vi "WPI_ADI_IMU_Open.vi"(8 "error in":errorcluster, 9 "AHRS Algorithm":enum16{"Complementary", "Madgwick"}(ring), 10 "Yaw Axis":enum16{"X", "Y", "Z"}(ring)=enum."Z", 11 "SPI Chip Select":T3=enum."SPI MXP") -> (0 "error out":errorcluster, 3 "ADI IMU Interrupt DevRef":T1={"SimpleGyroDevRef"={"DevStatus"={"status"=FALSE, "code"=0, "source"=""}, "Handle"=0, "SPI Bus"=enum."SPI On-Board, CS0", "Device Found"=FALSE, "Sample Rate"=0.0, "Device Ready"=FALSE, "Yaw Axis"=enum."Z", "AHRS Algorithm"=enum."Complementary"}, "InterruptRef"={"DevStatus"={"status"=FALSE, "code"=0, "source"=""}, "InterruptIndex"=enum."0"}} {"SimpleGyroDevRef"."Sample Rate" min=0.25 max=100.0 step=0.25})   [LabVIEW 2015, in "FRC ADI MXP IMU.lvlib"]
doc: "Initiates communication between an Analog Devices MXP IMU and the RoboRIO."
uses:
  FRC ADI MXP IMU.lvlib
  <vilib>/Rock Robotics/SystemInterfaces/spilib/spi_bus.ctl
  WPI_AnalogDevicesIMUInterruptDevRef.ctl
  WPI_AnalogDevicesIMUDevRef.ctl
  <vilib>/Rock Robotics/WPI/Interrupt/WPI_InterruptRef.ctl
  <vilib>/Rock Robotics/SystemInterfaces/Interrupt/FPGA_InterruptIndex.ctl
  <vilib>/Rock Robotics/WPI/SPI/WPI_SPIMode.ctl
  <vilib>/Rock Robotics/SystemInterfaces/DIO/FPGA_DIOChannel.ctl
  WPI_IMU_ADIS16448_Registers.ctl
  <vilib>/Rock Robotics/WPI/Counter/WPI_CounterDigitalInputToDigitalSource.vi
  <vilib>/Rock Robotics/SystemInterfaces/CounterEncoderSourceConvertion/FPGA_CounterEncoderSourceConvertionLVSourceTypeToFPGAType.vi
  <vilib>/Rock Robotics/WPI/Interrupt/WPI_InterruptCache.vi
  <vilib>/Rock Robotics/SystemInterfaces/Interrupt/FPGA_InterruptWriteConfiguration.vi
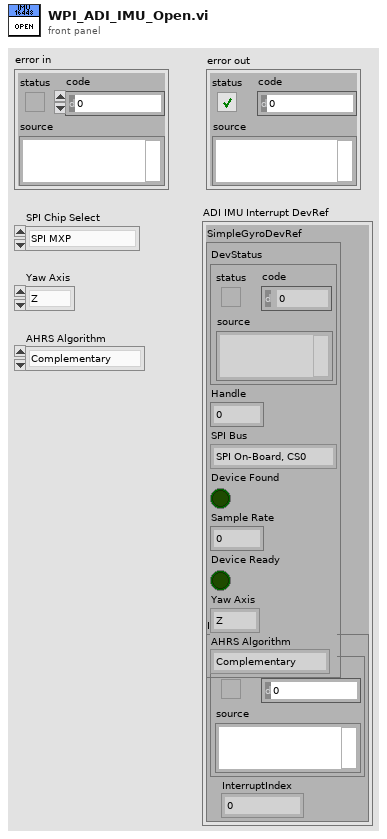
[diagram p1: front panel]
types:
  T1 = typedef "FRC ADI MXP IMU.lvlib/WPI_AnalogDevicesIMUInterruptDevRef.ctl" = cluster{"SimpleGyroDevRef":T2, "InterruptRef":T4}
  T2 = typedef "FRC ADI MXP IMU.lvlib/WPI_AnalogDevicesIMUDevRef.ctl" = cluster{"DevStatus":errorcluster, "Handle":i32, "SPI Bus":T3, "Device Found":bool, "Sample Rate":dbl, "Device Ready":bool, "Yaw Axis":enum16{"X", "Y", "Z"}, "AHRS Algorithm":enum16{"Complementary", "Madgwick"}}
  T3 = typedef "spi_bus.ctl" = enum16{"SPI On-Board, CS0", "SPI On-Board, CS1", "SPI On-Board, CS2", "SPI On-Board, CS3", "SPI MXP", "Invalid"}
  T4 = typedef "WPI_InterruptRef.ctl" = cluster{"DevStatus":errorcluster, "InterruptIndex":T5}
  T5 = typedef "FPGA_InterruptIndex.ctl" = enum8{"0", "1", "2", "3", "4", "5", "6", "7", "Invalid"}
  T6 = typedef "FPGA_DIOChannel.ctl" = enum8{"DIO 0", "DIO 1", "DIO 2", "DIO 3", "DIO 4", "DIO 5", "DIO 6", "DIO 7", "DIO 8", "DIO 9", "DIO MXP 0", "DIO MXP 1", "DIO MXP 2", "DIO MXP 3", "DIO MXP 4", "DIO MXP 5", "DIO MXP 6", "DIO MXP 7", "DIO MXP 8", "DIO MXP 9", "DIO MXP 10", "DIO MXP 11", "DIO MXP 12", "DIO MXP 13", "DIO MXP 14", "DIO MXP 15", "Invalid"}
  T7 = typedef "WPI_SPIMode.ctl" = enum16{"Mode 0 (Clk Idle Low,Sample on Leading)", "Mode 1 (Clk Idle Low,Sample on Trailing)", "Mode 2 (Clk Idle High,Sample on Leading)", "Mode 3 (Clk Idle High,Sample on Trailing)"}
  T8 = typedef "FRC ADI MXP IMU.lvlib/WPI_IMU_ADIS16448_Registers.ctl" = u8
  T9 = typedef "WPI_SPIDevRef.ctl" = cluster{"DevStatus":errorcluster, "Handle":i32, "SPI Bus":T3}
  T10 = typedef "WPI_DigitalInputDevRef.ctl" = cluster{"DevStatus":errorcluster, "DIO Channel":T6}
  T11 = typedef "FPGA_CounterEncoderSourceConvertionLVSourceType.ctl" = cluster{"DevStatus":errorcluster, "AnalogTriggerMode?":bool, "DigitalMode":cluster{"DIO Channel":T12}, "AnalogTriggerMode":cluster{"AnalogTriggerIndex":T13, "OutputType":T14}}
  T12 = typedef "FPGA_DIODigitalSourceChannel.ctl" = enum8{"DIO 0", "DIO 1", "DIO 2", "DIO 3", "DIO 4", "DIO 5", "DIO 6", "DIO 7", "DIO 8", "DIO 9", "DIO MXP 0", "DIO MXP 1", "DIO MXP 2", "DIO MXP 3", "DIO MXP 4", "DIO MXP 5", "DIO MXP 6", "DIO MXP 7", "DIO MXP 8", "DIO MXP 9", "DIO MXP 10", "DIO MXP 11", "DIO MXP 12", "DIO MXP 13", "DIO MXP 14", "DIO MXP 15", "Disabled"}
  T13 = typedef "FPGA_AnalogTriggerIndex.ctl" = enum8{"Trig 0", "Trig 1", "Trig 2", "Trig 3", "Trig 4", "Trig 5", "Trig 6", "Trig 7", "Invalid"}
  T14 = typedef "FPGA_AnalogTriggerOutType.ctl" = enum16{"InWindow", "TriggerState", "Rising", "Falling"}
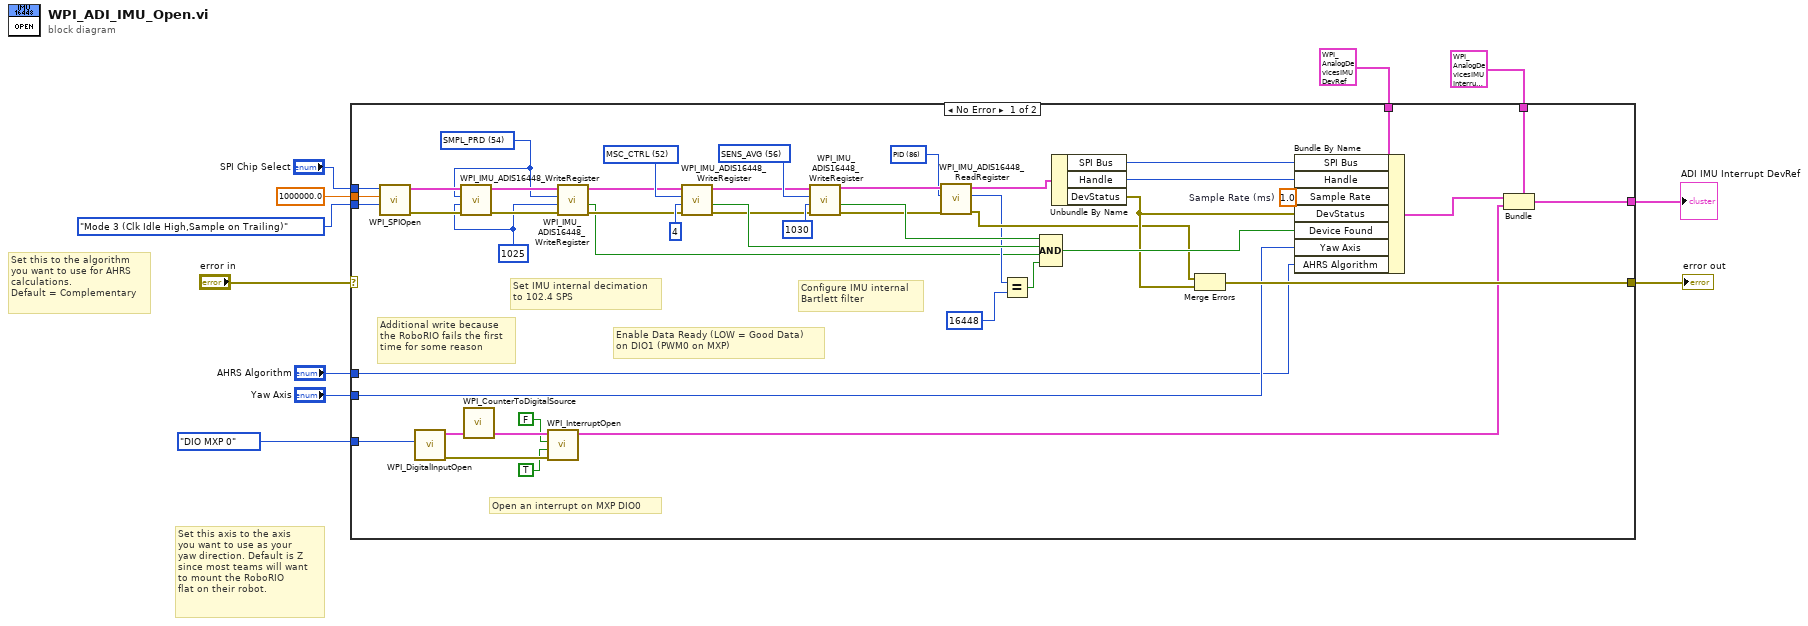
[diagram p0: block diagram]
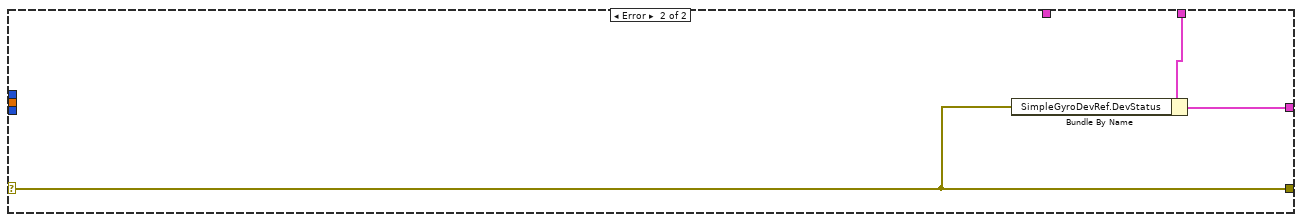
[diagram p2: hidden frame]
diagram:
  # "Set this to the algorithm\nyou want to use for AHRS\ncalculations. \nDefault = Complementary"
  # "Set this axis to the axis\nyou want to use as your\nyaw direction. Default is Z\nsince most teams will want \nto mount the RoboRIO\nflat on their robot."
  n1 = case shown="No Error" "error in" {
    selector: "error in" -> [_ w60]
    tunnel: "SPI Chip Select" -> [w58 _]
    tunnel: 1000000.0 ("Clock Rate (Hz)") -> [w57 _]
    tunnel: WPI_SPIMode."Mode 3 (Clk Idle High,Sample on Trailing)" ("Mode (3)") -> [w56 _]
    tunnel: [w46 w60] -> w7
    tunnel: T2 {"DevStatus"={"status"=FALSE, "code"=0, "source"=""}, "Handle"=0, "SPI Bus"=enum."SPI On-Board, CS0", "Device Found"=FALSE, "Sample Rate"=0.0, "Device Ready"=FALSE, "Yaw Axis"=enum."Z", "AHRS Algorithm"=enum."Complementary"} ("SimpleGyroDevRef 2") -> [w55 _]
    tunnel: [w33 w59] -> w3
    tunnel: T1 {"SimpleGyroDevRef"={"DevStatus"={"status"=FALSE, "code"=0, "source"=""}, "Handle"=0, "SPI Bus"=enum."SPI On-Board, CS0", "Device Found"=FALSE, "Sample Rate"=0.0, "Device Ready"=FALSE, "Yaw Axis"=enum."Z", "AHRS Algorithm"=enum."Complementary"}, "InterruptRef"={"DevStatus"={"status"=FALSE, "code"=0, "source"=""}, "InterruptIndex"=enum."0"}} ("output cluster") -> [w32 w61]
    tunnel: FPGA_DIOChannel."DIO MXP 0" ("DIO Channel") -> [w31 _]
    tunnel: "Yaw Axis" -> [w13 _]
    tunnel: "AHRS Algorithm" -> [w12 _]
    frame No Error {
      w27 = T8 86 items=["SMPL_PRD"=54, "SENS_AVG"=56, "MSC_CTRL"=52, "ERROR_FLAGS"=60, "TEMP"=44, "BARO"=40, "Z_MAG"=36, "Y_MAG"=32, "X_MAG"=28, "Z_ACCEL"=24, "Y_ACCEL"=20, "X_ACCEL"=16, "Z_GYRO"=12, "Y_GYRO"=8, "X_GYRO"=4, "PID"=86] ("ADIS16448 Register")
      w52 = 1.0  # Sample Rate (ms)
      w45 = T8 56 items=["SMPL_PRD"=54, "SENS_AVG"=56, "MSC_CTRL"=52, "ERROR_FLAGS"=60, "TEMP"=44, "BARO"=40, "Z_MAG"=36, "Y_MAG"=32, "X_MAG"=28, "Z_ACCEL"=24, "Y_ACCEL"=20, "X_ACCEL"=16, "Z_GYRO"=12, "Y_GYRO"=8, "X_GYRO"=4, "PID"=86] ("ADIS16448 Register")
      w51 = T8 52 items=["SMPL_PRD"=54, "SENS_AVG"=56, "MSC_CTRL"=52, "ERROR_FLAGS"=60, "TEMP"=44, "BARO"=40, "Z_MAG"=36, "Y_MAG"=32, "X_MAG"=28, "Z_ACCEL"=24, "Y_ACCEL"=20, "X_ACCEL"=16, "Z_GYRO"=12, "Y_GYRO"=8, "X_GYRO"=4, "PID"=86] ("ADIS16448 Register")
      w17 = u16 1025 ("Data")
      w16 = T8 54 items=["SMPL_PRD"=54, "SENS_AVG"=56, "MSC_CTRL"=52, "ERROR_FLAGS"=60, "TEMP"=44, "BARO"=40, "Z_MAG"=36, "Y_MAG"=32, "X_MAG"=28, "Z_ACCEL"=24, "Y_ACCEL"=20, "X_ACCEL"=16, "Z_GYRO"=12, "Y_GYRO"=8, "X_GYRO"=4, "PID"=86] ("ADIS16448 Register")
      # "Open an interrupt on MXP DIO0"
      # "Additional write because\nthe RoboRIO fails the first\ntime for some reason"
      # "Configure IMU internal\nBartlett filter"
      # "Enable Data Ready (LOW = Good Data) \non DIO1 (PWM0 on MXP)"
      # "Set IMU internal decimation\nto 102.4 SPS"
      n2 = call <vilib>:"WPI_SPIOpen.vi"("Mode (3)"=w56, "Clock Rate (Hz)"=w57, "SPI Bus"=w58) -> ("error out"=w18:errorcluster, "SPIDevRef"=w21:T9)  [unwired: 7 in]
      n3 = call <vilib>:"WPI_DigitalInputOpen.vi"("DIO Channel"=w31) -> ("error out"=w38:errorcluster, "DigitalInputDevRef"=w40:T10)  [unwired: 9 in]
      n4 = call "WPI_IMU_ADIS16448_WriteRegister.vi"("error in (no error)"=w18, "Data"=w17, "ADIS16448 Register"=w16, "SPIDevRef in"=w21) -> ("error out"=w19:errorcluster, "SPIDevRef out"=w20:T9)  [unwired: 4 in, 2 out]
      n5 = call-poly <vilib>:"WPI_CounterToDigitalSource.vi"("DigitalInputDevRef"=w40) -> ("Digital Source"=w39:T11)  [unwired: 6 in]
      n6 = call <vilib>:"WPI_InterruptOpen.vi"("error in (no error)"=w38, "Falling Edge"=TRUE, "Rising Edge"=FALSE, "Source"=w39) -> ("InterruptRef"=w35:T4)  [unwired: 6 in, 1 out]
      n7 = call "WPI_IMU_ADIS16448_WriteRegister.vi"("error in (no error)"=w19, "Data"=w17, "ADIS16448 Register"=w16, "SPIDevRef in"=w20) -> ("error out"=w24:errorcluster, "Write OK?"=w14:bool, "SPIDevRef out"=w25:T9)  [unwired: 4 in, 1 out]
      n8 = call "WPI_IMU_ADIS16448_WriteRegister.vi"("error in (no error)"=w24, "Data"=u16 4, "ADIS16448 Register"=w51, "SPIDevRef in"=w25) -> ("error out"=w42:errorcluster, "Write OK?"=w48:bool, "SPIDevRef out"=w43:T9)  [unwired: 4 in, 1 out]
      n9 = call "WPI_IMU_ADIS16448_WriteRegister.vi"("error in (no error)"=w42, "Data"=u16 1030, "ADIS16448 Register"=w45, "SPIDevRef in"=w43) -> ("error out"=w28:errorcluster, "Write OK?"=w41:bool, "SPIDevRef out"=w29:T9)  [unwired: 4 in, 1 out]
      n10 = call "WPI_IMU_ADIS16448_ReadRegister.vi"("error in (no error)"=w28, "Register"=w27, "SPIDevRef in"=w29) -> ("error out"=w26:errorcluster, "Register Value"=w23:u16, "SPIDevRef out"=w30:T9)  [unwired: 6 in]
      n11 = Equal?(x=w23, y=u16 16448) -> (x = y?=w15:bool)
      n12 = Compound Arithmetic op=AND(w41, w48, w14, w15) -> (w49:bool)
      n13 = Unbundle By Name(w30) -> ("SPI Bus"=w54:T3, "Handle"=w53:i32, "DevStatus"=w47:errorcluster)
      n14 = Merge Errors(w26, w47) -> (w46:errorcluster)
      n15 = Bundle By Name(cluster=w55, "SPI Bus"=w54, "Handle"=w53, "Sample Rate"=w52, "DevStatus"=w47, "Device Found"=w49, "Yaw Axis"=w13, "AHRS Algorithm"=w12) -> (w34:T2)
      n16 = Bundle(cluster=w32, "SimpleGyroDevRef"=w34, "InterruptRef"=w35) -> (w33:T1)
    }
    frame Error {
      n17 = Bundle By Name(cluster=w61, "SimpleGyroDevRef.DevStatus"=w60) -> (w59:T1)
    }
  }
  "error out" <- w7
  "ADI IMU Interrupt DevRef" <- w3
